vi "Get Data and Log.vi"() -> ()   [LabVIEW 2016]
uses:
  <vilib>/Rock Robotics/Network Tables/NT Read Numeric Array.vi
  <vilib>/Utility/file.llb/Write Delimited Spreadsheet (DBL).vi
panel:
  in  "Mode":T1(ring)=enum."Auto Disabled"
  out "appended path":path
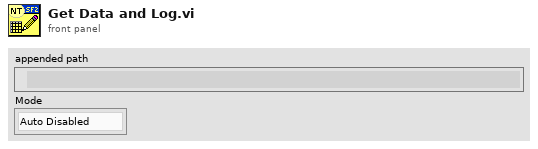
[diagram p1: front panel]
types:
  T1 = enum8{"Tele-Op Disabled", "Tele-Op Enabled", "Auto Disabled", "Auto Enabled", "Test Disabled", "Test Enabled", "Disconnected", "No Code", "E-Stop"}
  T2 = enum16{"open", "replace", "create", "open or create", "replace or create", "replace or create with confirmation"}
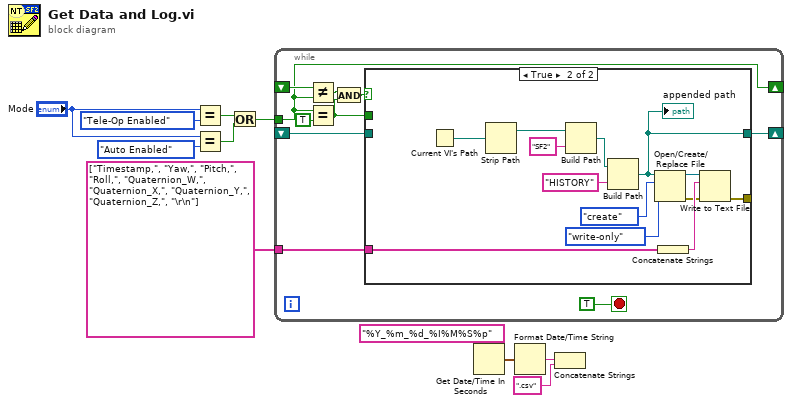
[diagram p0: block diagram]
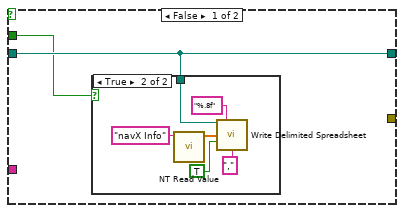
[diagram p2: hidden frame]
diagram:
  (unwired) "%Y_%m_%d_%I%M%S%p" ("time format string (%c)")
  n1 = Equal?(x="Mode", y=T1."Tele-Op Enabled") -> (x = y?=w7:bool)
  n2 = Equal?(x="Mode", y=T1."Auto Enabled") -> (x = y?=w6:bool)
  n3 = Or(x=w7, y=w6) -> (x .or. y?=w5:bool)
  n4 = while {
    shift-right: [w18] -> _
    shift-left: _ -> [w19]
    tunnel: w5 -> [w15]
    shift-right: [w15] -> _
    shift-left: _ -> [w17]
    tunnel: string[] ["Timestamp,", "Yaw,", "Pitch,", "Roll,", "Quaternion_W,", "Quaternion_X,", "Quaternion_Y,", "Quaternion_Z,", "\r\n"] -> [w11]
    stop <- TRUE stop-if-true
    n5 = Not Equal?(x=w17, y=w15) -> (x != y?=w16:bool)
    n6 = Equal?(x=w15, y=TRUE) -> (x = y?=w12:bool)
    n7 = And(x=w16, y=w12) -> (x .and. y?=w13:bool)
    n8 = case shown="True" w13 {
      tunnel: [w22 w35] -> w18
      tunnel: w19 -> [w22 _]
      tunnel: w12 -> [w21 _]
      tunnel: w11 -> [_ w37]
      tunnel: [_ w31] -> _
      frame False {
        n9 = case shown="True" w21 {
          tunnel: w22 -> [_ w25]
          frame False {
          }
          frame True {
            n10 = call-poly <vilib>:"NT Read Value.vi"("Name"="navX Info") -> ("Numeric Array"=w24:dbl[])  [unwired: 9 in, 1 out]
            n11 = call-poly <vilib>:"Write Delimited Spreadsheet.vi"("file path (dialog if empty)"=w25, "format (%.3f)"="%.8f", "1D data"=w24, "append to file? (new file:F)"=TRUE, "delimiter (\\t)"="," ("delimiter (\\t)")) -> ()  [unwired: 9 in, 2 out]
          }
        }
      }
      frame True {
        n12 = Current VI's Path() -> (path=w34:path)
        n13 = Strip Path(path=w34) -> (stripped path=w33:path)  [unwired: 1 out]
        n14 = Build Path(base path=w33, name or relative path="SF2") -> (appended path=w38:path)
        n15 = Build Path(base path=w38, name or relative path="HISTORY") -> (appended path=w35:path)
        "appended path" <- w35
        n16 = Open/Create/Replace File(file path (use dialog)=w35, operation (0:open)=T2."create", access (0:read/write)=enum16{"read/write", "read-only", "write-only"}."write-only") -> (refnum out=w41:refnum<file>, error out=w32:errorcluster)  [unwired: 3 in, 1 out]
        n17 = Concatenate Strings(w37) -> (w36:string)
        n18 = Write to Text File(file (use dialog)=w41, text=w36, error in=w32) -> (error out=w31:errorcluster)  [unwired: 1 in, 2 out]
      }
    }
  }
  n19 = Get Date/Time In Seconds() -> (seconds since 1Jan1904=w1:timestamp)
  n20 = Format Date/Time String(seconds (now)=w1) -> (date/time string=w2:string)  [unwired: 2 in]
  n21 = Concatenate Strings(w2, ".csv" ("string")) -> ()  [unwired: 1 out]
